vi "Determine_Save_Order.vi"(8 "error in (no error)":errorcluster, 10 "all VIs in memory":string[](array[string]), 11 "AB_Source_VI in":refnum<class "AB_Source_VI.lvclass">) -> (0 "error out":errorcluster, 2 "saveOrder":i32, 3 "AB_Source_VI out":refnum<class "AB_Source_VI.lvclass">)   [LabVIEW 2020, in "AB_Source_VI.lvclass"]
uses:
  <vilib>/AppBuilder/AB_Classes/Source/VI/AB_Source_VI.lvclass
  e:/builds/penguin/labview/branches/2020/dev/dist/vi.lib/AppBuilder/AB_Classes/Source/AB_Source.lvclass
  <vilib>/AppBuilder/AB_Classes/Source/AB_Source.lvclass
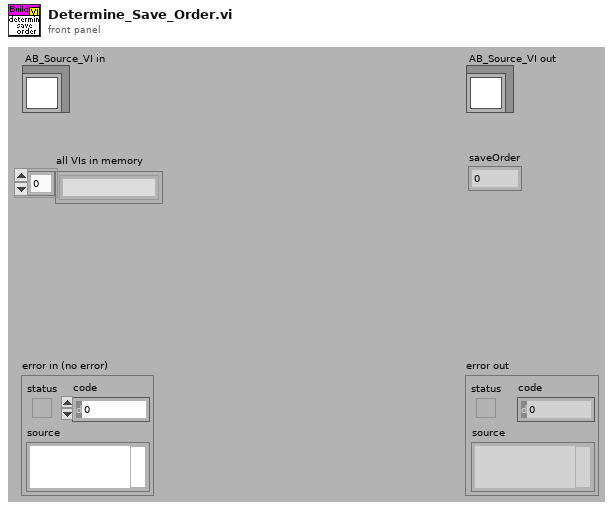
[diagram p1: front panel]
types:
  T1 = typedef "AB_Source.ctl" = cluster{"path":path, "itemID":string, "parentIndex":i32, "sourceInclusion":T2, "destinationIndex":i32, "properties":T3[], "newName":string, "lvfile":bool, "valid":bool, "eng_inBuild":bool, "eng_isNonVILink":bool, "Amalgamation":bool, "Amalgamation Piece":bool, "eng_delimitedName":string, "preventRename":bool}
  T2 = typedef "AB_Source_Inclusion.ctl" = enum16{"IncludeIfReferenced", "Include", "Exclude", "TopLevel"}
  T3 = typedef "AB_Source_Properties.ctl" = cluster{"sourcePropertyType":T4, "value":variant}
  T4 = typedef "AB_Source_Property_Type.ctl" = enum16{"Remove block diagram", "Remove front panel", "Password", "Window has title bar", "Show menu bar", "Show vertical scroll bar", "Show horizontal scroll bar", "Show toolbar", "Show Abort button", "Show fp when called", "Window behavior", "Allow user to close window", "Window run-time position", "Run when opened", "Allow debugging", "Auto error handling", "Generate guard code", "Use stack variables", "Expression folding", "Integer only", "Inline subVI"}
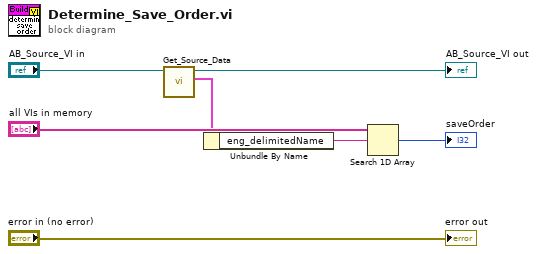
[diagram p0: block diagram]
diagram:
  n1 = call <vilib>:"Get_Source_Data.vi"("Class in"="AB_Source_VI in") -> ("data"=w1:T1, "Class out"=→"AB_Source_VI out":refnum<class "AB_Source_VI.lvclass">)  [unwired: 8 in, 1 out]
  n2 = Unbundle By Name(w1) -> ("eng_delimitedName"=w7:string)
  n3 = Search 1D Array(1D array="all VIs in memory", element=w7) -> (index of element=→"saveOrder":i32)  [unwired: 1 in]
  "error out" <- "error in (no error)"
